vi "Ejercicio_1_1.vi"() -> ()   [LabVIEW 2020]
panel:
  out "?":string="Guarda el valor hasta que se vuelve a pulsar."
  out "?":string="Cambia el valor cuando deja recibir el pulso y se regresa a su estado inicial."
  out "?":string="Cambia el valor cuando recibe el pulso y guarda el nuevo."
  out "?":string="El LED enciende mientras pulsas."
  out "?":string="En cuanto se suelta, el LED enciende."
  out "?":string="En cuanto se presiona, el LED enciende."
  out "LED 6":bool
  out "LED 5":bool
  out "LED 4":bool
  out "LED 3":bool
  out "LED 2":bool
  out "LED 1":bool
  in  "Boton 6":bool
  in  "Boton 5":bool
  in  "Boton 4":bool
  in  "Boton 3":bool
  in  "Boton 2":bool
  in  "Boton 1":bool
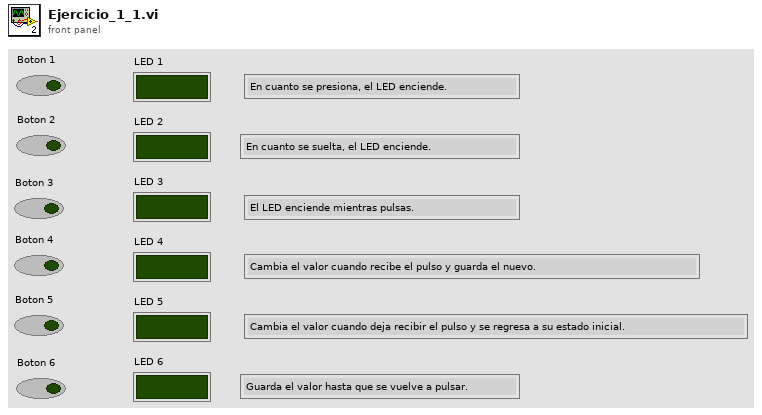
[diagram p1: front panel]
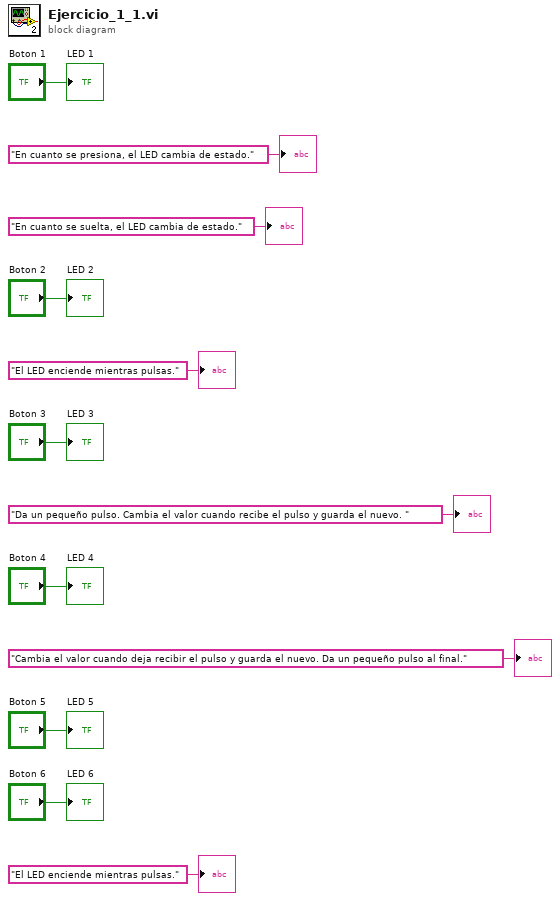
[diagram p0: block diagram]
diagram:
  "LED 1" <- "Boton 1"
  "LED 2" <- "Boton 2"
  "LED 3" <- "Boton 3"
  "LED 4" <- "Boton 4"
  "LED 5" <- "Boton 5"
  "LED 6" <- "Boton 6"
  "?" <- "En cuanto se presiona, el LED cambia de estado."
  "?" <- "En cuanto se suelta, el LED cambia de estado."
  "?" <- "El LED enciende mientras pulsas."
  "?" <- "Da un pequeño pulso. Cambia el valor cuando recibe el pulso y guarda el nuevo. "
  "?" <- "Cambia el valor cuando deja recibir el pulso y guarda el nuevo. Da un pequeño pulso al final."
  "?" <- "El LED enciende mientras pulsas."
